vi "Write Peaks to Excel sheet.vi"(6 "action":enum16{"open", "append", "close"}(ring)=enum."append", 8 "error in (no error)":errorcluster, 11 "Peaks":T1(array[cluster]) {"Area" format="%.4f"; "Summit Y" format="%.4f"; "End Y" format="%.4f"; "End X" format="%.4f"; "Summit X" format="%.4f"; "Start Y" format="%.4f"; "Start X" format="%.4f"}) -> (0 "error out":errorcluster)   [LabVIEW 2012]
doc: "This VI demonstrates the basic idea of using the OLE Automation VIs by writing a Table into an Excel WorkSheet."
panel:
  out "row":i32
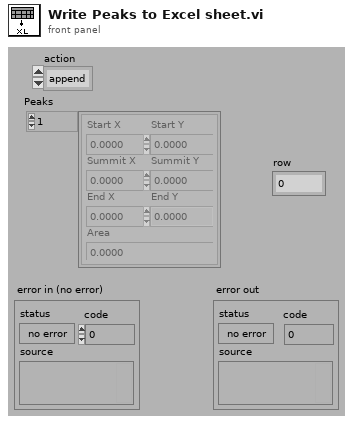
[diagram p1: front panel]
types:
  T1 = cluster{"Start X":dbl, "Start Y":dbl, "Summit X":dbl, "Summit Y":dbl, "End X":dbl, "End Y":dbl, "Area":dbl}[]
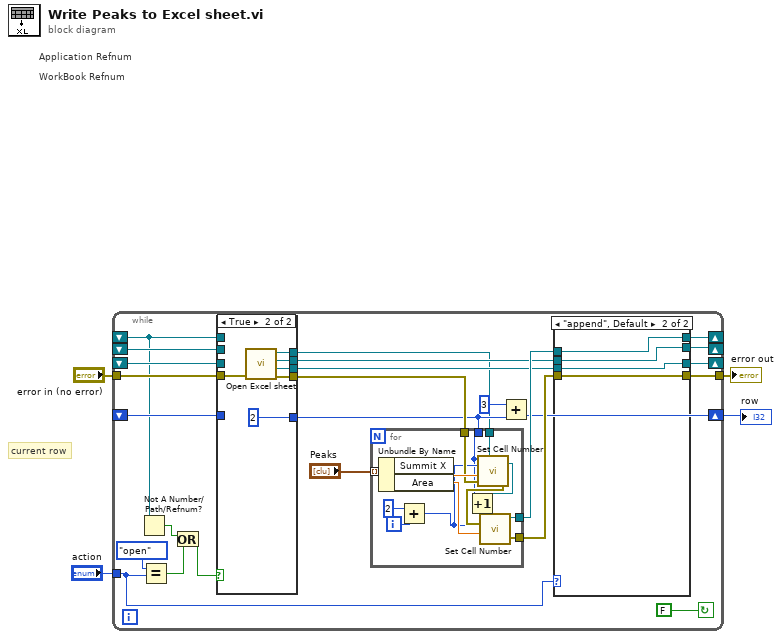
[diagram p0: block diagram]
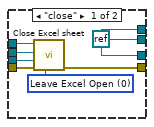
[diagram p2: hidden frame]
diagram:
  # "current row"
  # "WorkBook Refnum"
  # "Application Refnum"
  n1 = while {
    shift-left: _ -> [w16]
    shift-right: [w18] -> _
    shift-left: _ -> [w17]
    shift-right: [w19] -> _
    shift-left: _ -> [w11]
    shift-right: [w20] -> _
    tunnel: [w21] -> w2
    tunnel: "error in (no error)" -> [w27]
    tunnel: "action" -> [w10]
    shift-left: _ -> [w12]
    shift-right: [w13] -> w1
    stop <- FALSE continue-if-true
    n2 = Not A Number/Path/Refnum?(number/path/refnum=w11) -> (NaN/Path/Refnum?=w8:bool)
    n3 = Equal?(x=enum16{"open", "append", "close"}."open", y=w10) -> (x = y?=w7:bool)
    n4 = Or(x=w8, y=w7) -> (x .or. y?=w6:bool)
    n5 = case shown="True" w6 {
      tunnel: w27 -> [w42 w51]
      tunnel: [w45 w50] -> w5
      tunnel: [w44 w49] -> w25
      tunnel: [w43 w48] -> w24
      tunnel: [w42 w47] -> w23
      tunnel: w11 -> [w45 _]
      tunnel: w17 -> [w44 _]
      tunnel: w16 -> [w43 _]
      tunnel: [w41 2] -> w15
      tunnel: w12 -> [w41 _]
      frame False {
      }
      frame True {
        n6 = call "Open Excel sheet.vi"("error in (no error)"=w51) -> ("error out"=w47:errorcluster, "Excel._Application"=w48:refnum<k7>, "Excel._Workbook"=w49:refnum<k7>, "Excel._Worksheet"=w50:refnum<k7>)  [unwired: 5 in]
      }
    }
    n7 = for {
      tunnel: "Peaks" -> [w65] mode=indexing
      tunnel: w5 -> [w62]
      tunnel: [w60] -> w26
      tunnel: w23 -> [w59]
      tunnel: [w57] -> w22
      tunnel: w15 -> [w53]
      i -> [w56]
      n8 = Unbundle By Name(w65) -> ("Summit X"=w64:dbl, "Area"=w63:dbl)
      n9 = Add(x=2, y=w56) -> (x+y=w54:i32)
      n10 = Increment(x=w53) -> (x+1=w52:i32)
      n11 = call "Set Cell Number.vi"("Row"=w53, "Col"=w54, "Value"=w64, "error in (no error)"=w59, "Excel._Worksheet"=w62) -> ("Excel._Worksheet"=w61:refnum<k7>, "error out"=w58:errorcluster)
      n12 = call "Set Cell Number.vi"("Row"=w52, "Col"=w54, "Value"=w63, "error in (no error)"=w58, "Excel._Worksheet"=w61) -> ("Excel._Worksheet"=w60:refnum<k7>, "error out"=w57:errorcluster)
    }
    n13 = Add(x=3, y=w15) -> (x+y=w13:i32)
    n14 = case shown="\"append\", Default" w10 {
      tunnel: w26 -> [w36 w40]
      tunnel: w25 -> [w35 w39]
      tunnel: w24 -> [w34 w38]
      tunnel: w22 -> [w33 w37]
      tunnel: [w32 w37] -> w21
      tunnel: [w31 w40] -> w20
      tunnel: [w31 w39] -> w19
      tunnel: [w31 w38] -> w18
      frame "close" {
        w30 = u16 0 items=["Leave Excel Open", "Close Spreadsheet"] ("Completion Task")
        w31 = refnum<k0> refnum
        n15 = call "Close Excel sheet.vi"("Completion Task"=w30, "error out 2"=w33, "Excel._Application"=w34, "Excel._Workbook"=w35, "Excel._Worksheet"=w36) -> ("error out"=w32:errorcluster)  [unwired: 5 in]
      }
      frame "append", Default {
      }
    }
  }
  "error out" <- w2
  "row" <- w1
